vi "cvi_parse_records.vi"(8 "error in (no error)":errorcluster, 9 "tmode":u8=2, 10 "device":u8, 11 "fifo_buffer":u32[](array[numeric])) -> (0 "error out":errorcluster, 1 "channels":u8[](array[numeric]), 2 "sync":dbl[](array[numeric]), 3 "times":dbl[](array[numeric]))   [LabVIEW 2015]
uses:
  cvibuild.corr_funcs/Release/corr_funcs.dll
panel:
  # "device:\n0 - hydraharp\n1 - picoharp\n\ntmode:\n2 - T2\n3 - T3"
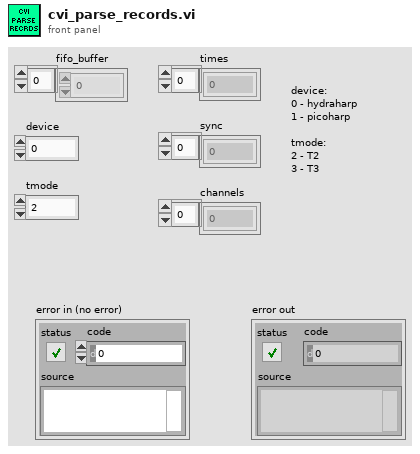
[diagram p1: front panel]
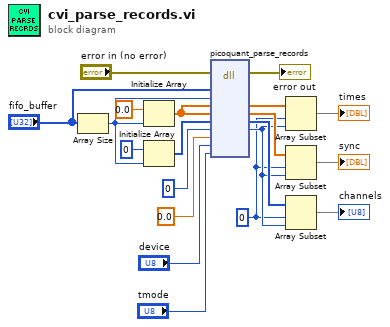
[diagram p0: block diagram]
diagram:
  w14 = 0 ("index")
  n1 = Array Size(array="fifo_buffer") -> (size(s)=w7:i32)
  n2 = Initialize Array(0.0 ("element"), w7) -> (w5:dbl[])
  n3 = Initialize Array(u8 0 ("element"), w7) -> (w8:u8[])
  n4 = dll-call lib="C:/Users/bspoka/Downloads/lvoop_dll-master/cvi_project/cvibuild.corr_funcs/Release/corr_funcs.dll" fn="picoquant_parse_records"(error in="error in (no error)", "fifo_buffer"="fifo_buffer", "fifo_size"=w7, "photon_times"=w5, "sync"=w5, "channels"=w8, "photon_count"=0, "overflow"=0.0, "device"="device", "tmode"="tmode") -> (error out=→"error out":errorcluster, "photon_times"=w13:dbl[], "sync"=w16:dbl[], "channels"=w17:u8[], "photon_count"=w15:i32)  [unwired: 8 in, 1 out]
  n5 = Array Subset(array=w13, index=w14, length=w15) -> (→"times":dbl[])
  n6 = Array Subset(array=w16, index=w14, length=w15) -> (→"sync":dbl[])
  n7 = Array Subset(array=w17, index=w14, length=w15) -> (→"channels":u8[])
